vi "TestExecuteBasicPolicy_PublishOK.vi"(8 "error in (no error)":errorcluster, 11 "TestCase in":refnum<class "TestSubscriptionPolicy.lvclass">) -> (0 "error out":errorcluster, 3 "TestCase out":refnum<class "TestSubscriptionPolicy.lvclass">)   [LabVIEW 2015, in "SubscriptionPolicy.lvlib" / "TestSubscriptionPolicy.lvclass"]
uses:
  TestSubscriptionPolicy.lvclass
  BasicSubscription/BasicSubscription.lvclass/BasicSubscription.ctl
  BasicSubscription/BasicSubscription.lvclass
  IMediator/ISubscriptionPolicy/ISubscriptionPolicy.lvclass
  Transport/QueueTransport/QueueTransport.lvclass
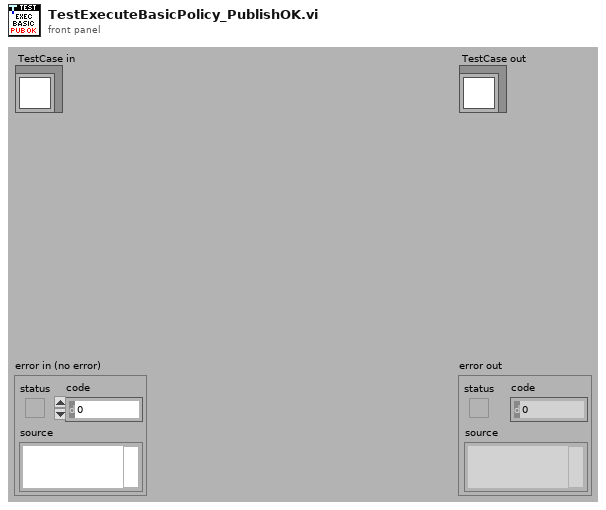
[diagram p1: front panel]
types:
  T1 = typedef "IMediator.lvlib/ISubscriptionPolicy.lvclass/ISubscriptionPolicy Reference.ctl" = refnum<data-value>
  T2 = cluster{"Data":variant, "Publication Time":timestamp}
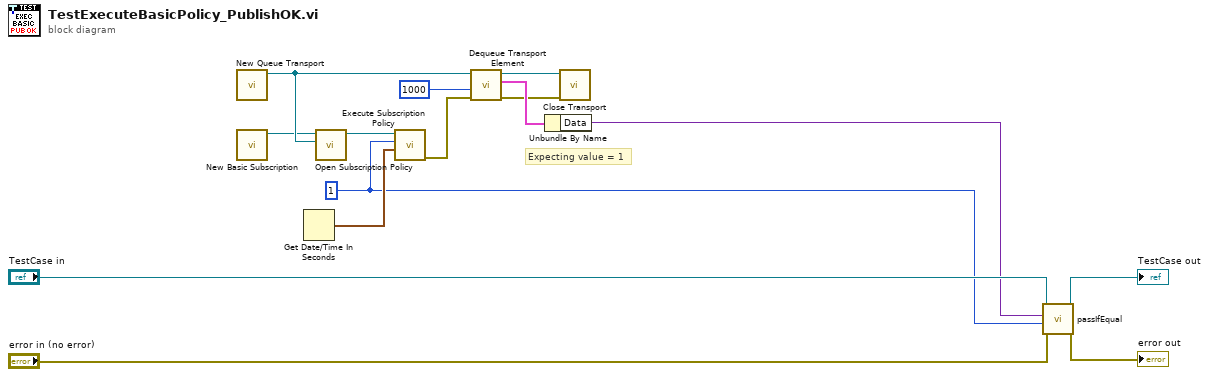
[diagram p0: block diagram]
diagram:
  w2 = 1
  # "Expecting value = 1"
  n1 = call "New Queue Transport.vi"() -> ("QueueTransport Out"=w10:refnum<class "QueueTransport.lvclass">)  [unwired: 10 in, 1 out]
  n2 = call "New Basic Subscription.vi"() -> ("BasicSubscription Out"=w1:refnum<class "BasicSubscription.lvclass">)  [unwired: 11 in]
  n3 = Get Date/Time In Seconds() -> (seconds since 1Jan1904=w6:timestamp)
  n4 = call "Open Subscription Policy.vi"("Transport"=w10, "SubscriptionPolicy"=w1) -> ("Subscription Policy"=w11:T1)  [unwired: 8 in, 1 out]
  n5 = call "Execute Subscription Policy.vi"("Publish Time"=w6, "New Topic Value"=w2, "Subscription Policy"=w11) -> ("error out (Unsubscribe?)"=w9:errorcluster)  [unwired: 8 in]
  n6 = call "Dequeue Transport Element.vi"("error in (no error)"=w9, "Timeout In ms (-1)"=1000, "QueueTransport in"=w10) -> ("error out"=w4:errorcluster, "Element"=w7:T2, "QueueTransport out"=w5:refnum<class "QueueTransport.lvclass">)  [unwired: 5 in, 1 out]
  n7 = Unbundle By Name(w7) -> ("Data"=w3:variant)
  n8 = call-dynamic "Close Transport.vi"("error in (no error)"=w4, "QueueTransport in"=w5) -> ()  [unwired: 9 in, 1 out]
  n9 = call-dynamic "passIfEqual.vi"("error in (no error)"="error in (no error)", "y"=w2, "x"=w3, "TestCase in"="TestCase in") -> ("error out"=→"error out":errorcluster, "TestCase out"=→"TestCase out":refnum<class "TestSubscriptionPolicy.lvclass">)  [unwired: 6 in]
